vi "_macro_Choreo_CommandDifferentialLTV.vi"() -> ()   [LabVIEW 2019, in "ChoreoLib.lvlib"]
uses:
  ChoreoLib.lvlib
  <vilib>/Rock Robotics/WPI/ThirdParty/JAS_Junk/TrajLib/TypeDef/POSE2D.ctl
  <vilib>/Rock Robotics/WPI/ThirdParty/JAS_Junk/TrajLib/TypeDef/TRANSLATION2D.ctl
  <vilib>/Rock Robotics/WPI/ThirdParty/JAS_Junk/TrajLib/TypeDef/ROTATION2D.ctl
  <vilib>/Rock Robotics/WPI/ThirdParty/JAS_Junk/TrajLib/VI/numCmd_Send_Generic.vi
  <vilib>/Rock Robotics/WPI/ThirdParty/JAS_Junk/TrajLib/VI/numCmd_ObtainQueue_Generic.vi
  <vilib>/Rock Robotics/WPI/ThirdParty/JAS_Junk/TrajLib/Trajectory_Library.lvlib
panel:
  in  "Initialize":bool
  in  "Current Position":T1={"TRANSLATION"={"X"=0.0, "Y"=0.0}, "ROTATION"={"VALUE"=0.0, "COS"=1.0, "SIN"=0.0}} {"ROTATION"."SIN" format="%13.4f"; "ROTATION"."COS" format="%13.4f"; "ROTATION"."VALUE" format="%13.4f"; "TRANSLATION"."Y" format="%14.3f"; "TRANSLATION"."X" format="%14.3f"}
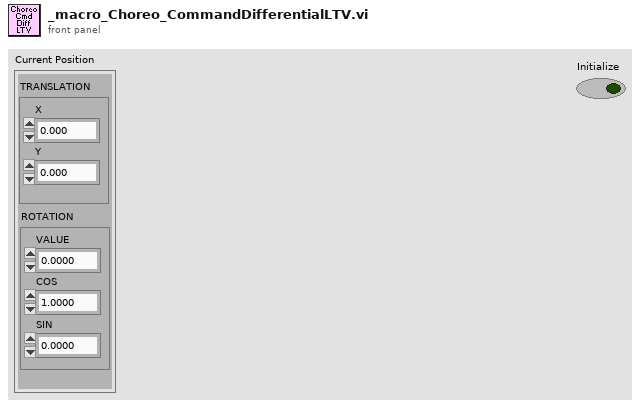
[diagram p1: front panel]
types:
  T1 = typedef "Trajectory_Library.lvlib/POSE2D.ctl" = cluster{"TRANSLATION":T2, "ROTATION":T3}
  T2 = typedef "Trajectory_Library.lvlib/TRANSLATION2D.ctl" = cluster{"X":dbl, "Y":dbl}
  T3 = typedef "Trajectory_Library.lvlib/ROTATION2D.ctl" = cluster{"VALUE":dbl, "COS":dbl, "SIN":dbl}
  T4 = typedef "Trajectory_Library.lvlib/CHASSIS_SPEEDS.ctl" = cluster{"vX":dbl, "vY":dbl, "vOmega":dbl}
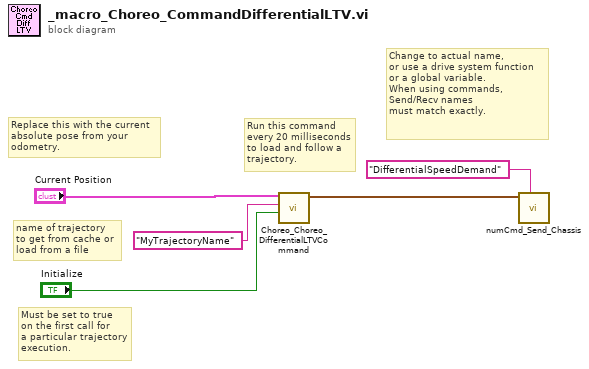
[diagram p0: block diagram]
diagram:
  # "Replace this with the current\nabsolute pose from your \nodometry."
  # "Run this command\nevery 20 milliseconds\nto load and follow a\ntrajectory."
  # "Must be set to true\non the first call for\na particular trajectory\nexecution."
  # "name of trajectory\nto get from cache or\nload from a file"
  # "Change to actual name, \nor use a drive system function\nor a global variable.  \nWhen using commands, \nSend/Recv names\nmust match exactly."
  n1 = call "Choreo_Choreo_DifferentialLTVCommand.vi"("Initialize"="Initialize", "TrajectoryName"="MyTrajectoryName", "Current Position"="Current Position") -> ("Chassis Speed Dmd"=w2:T4)  [unwired: 5 in, 3 out]
  n2 = call <vilib>:"numCmd_Send_Chassis.vi"("Command Name"="DifferentialSpeedDemand", "Chassis Speeds"=w2) -> ()  [unwired: 9 in, 1 out]
